vi "Flow Cal_Buffer_Dbl_VIG.vi"(0 "Fuel Temp":dbl, 1 "Operation":T4(ring)=enum."set raw data", 3 "Constants":cluster{"Ti":dbl, "SGi":dbl}, 5 "Calibration Formulas":T3, 9 "Flow (GPM)":dbl, 11 "error in":errorcluster, 12 "SGH20":dbl, 14 "Valid Flow Ranges":dbl[](array[numeric])) -> (4 "Addtional Values":T2, 6 "Current Formulas":T3, 10 "Calibrated Flow (lb/hr)":dbl, 15 "error out":errorcluster)   [LabVIEW 2018]
uses:
  Common/Controls/Parsed Formula TDEF.ctl
  <vilib>/gmath/NI_Gmath.lvlib
panel:
  in  "Calibration Info":T1
  out "Parsed Formula":cluster{"Table":i32[][], "Y Values":dbl[]}
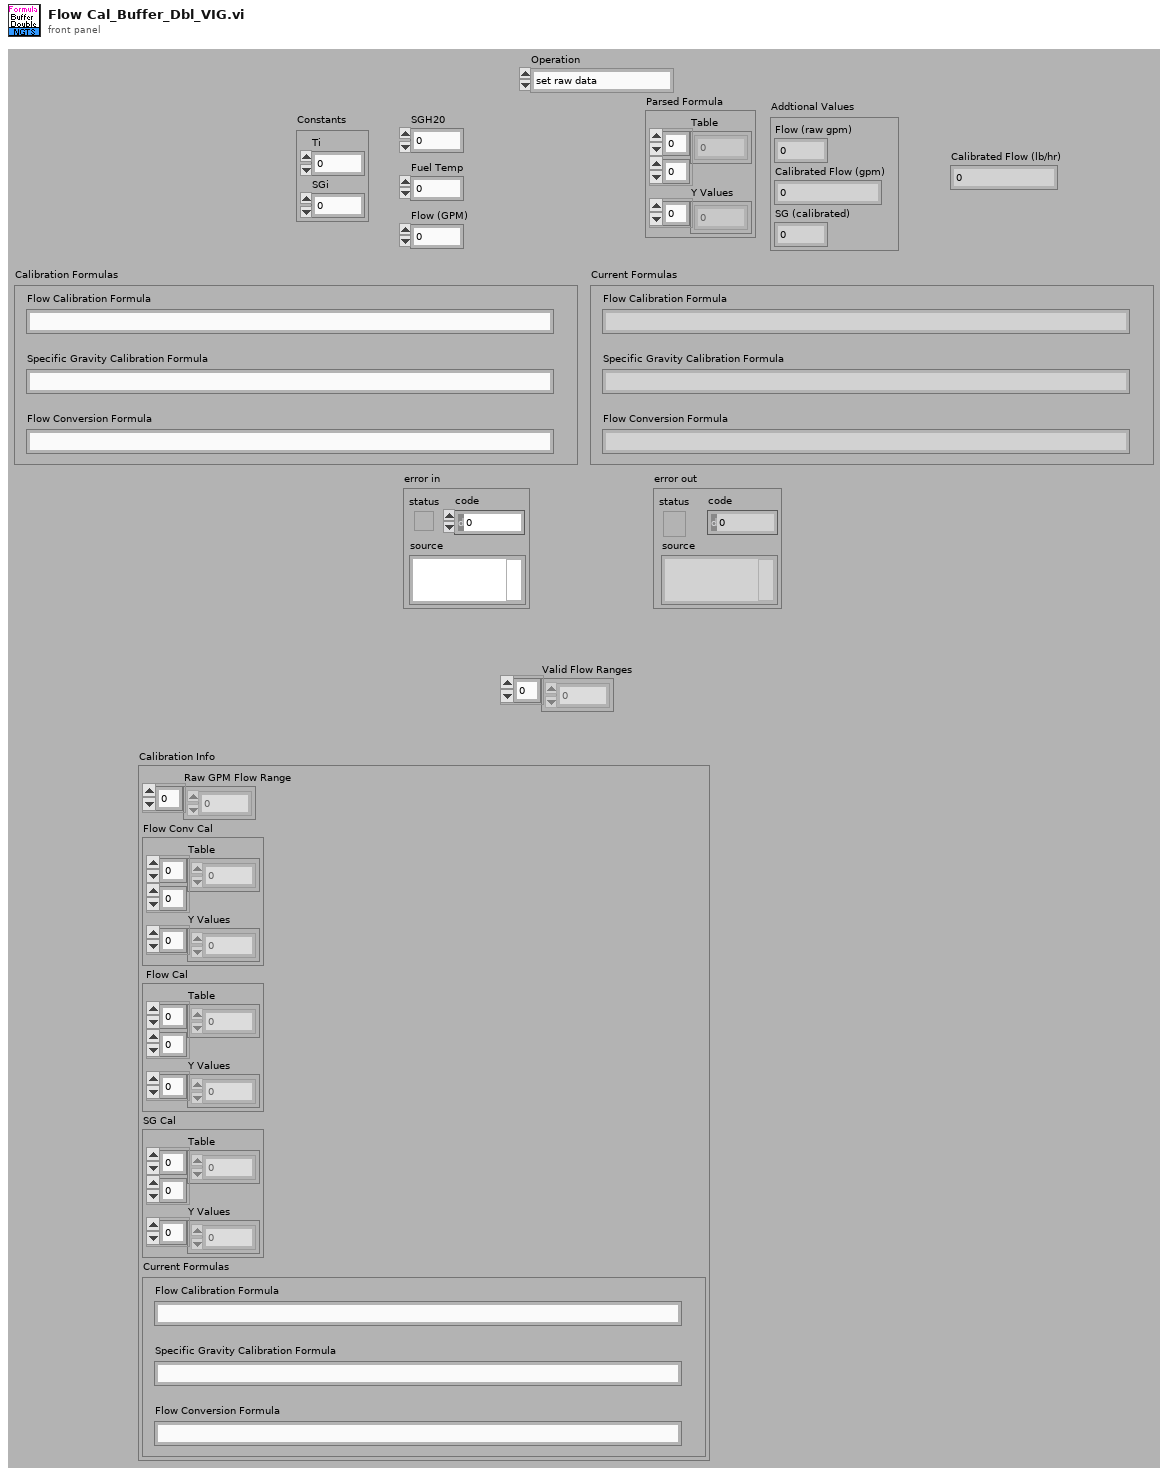
[diagram p1: front panel]
types:
  T1 = typedef "Parsed Formula TDEF.ctl" = cluster{"Raw GPM Flow Range":dbl[], "Flow Conv Cal":cluster{"Table":i32[][], "Y Values":dbl[]}, " Flow Cal":cluster{"Table":i32[][], "Y Values":dbl[]}, "SG Cal":cluster{"Table":i32[][], "Y Values":dbl[]}, "Current Formulas":cluster{"Flow Calibration Formula":string, "Specific Gravity Calibration Formula":string, "Flow Conversion Formula":string}}
  T2 = cluster{"Flow (raw gpm)":dbl, "Calibrated Flow (gpm)":dbl, "SG (calibrated)":dbl}
  T3 = cluster{"Flow Calibration Formula":string, "Specific Gravity Calibration Formula":string, "Flow Conversion Formula":string}
  T4 = enum16{"get data", "set raw data", "Set Ti and SGi and SGH20", "Add New Formula", "Get Formula", "initialize"}
  T5 = cluster{"element":dbl, "Flow (GPM)":dbl, "y value":dbl}
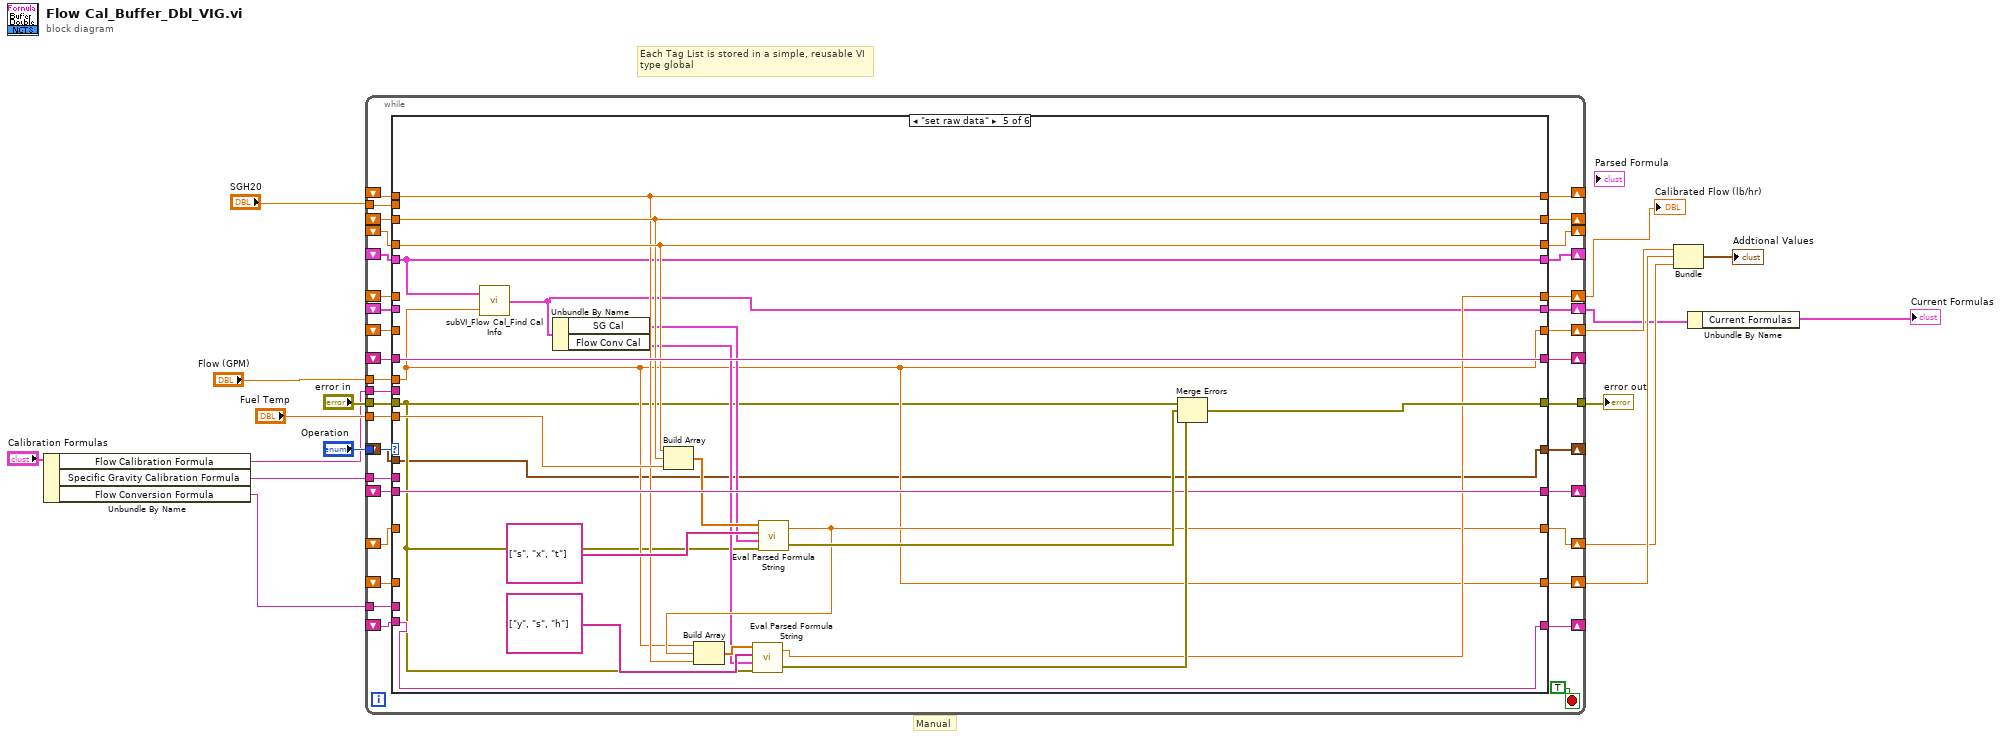
[diagram p0: block diagram]
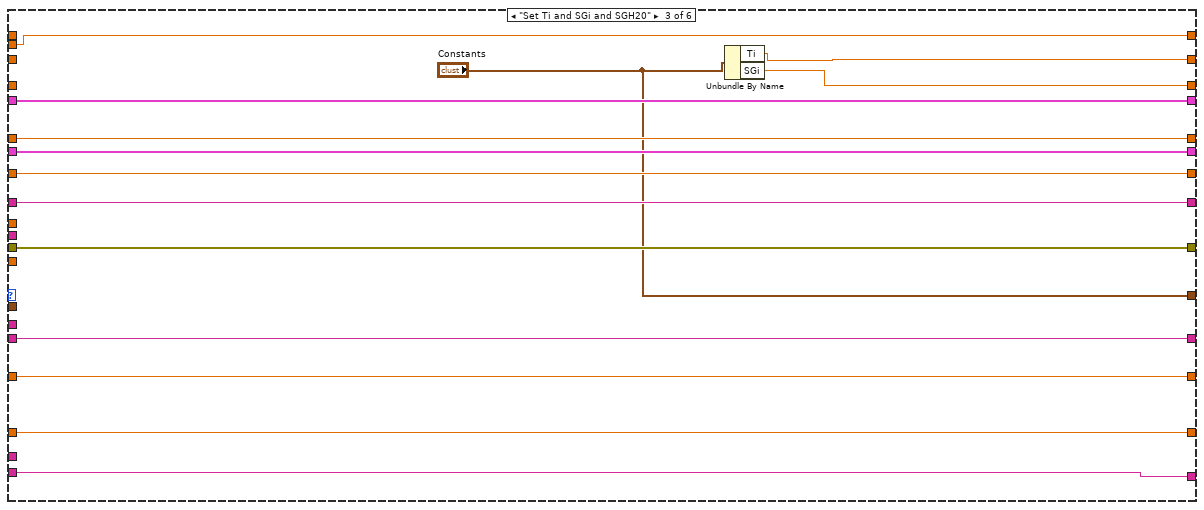
[diagram p4: hidden frame]
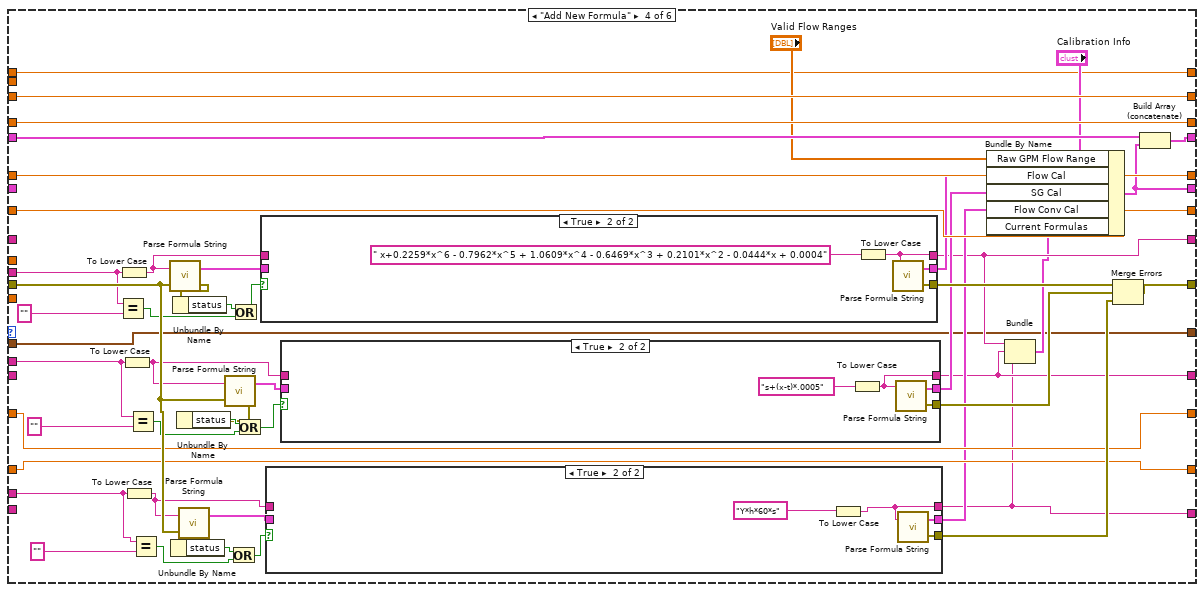
[diagram p5: hidden frame]
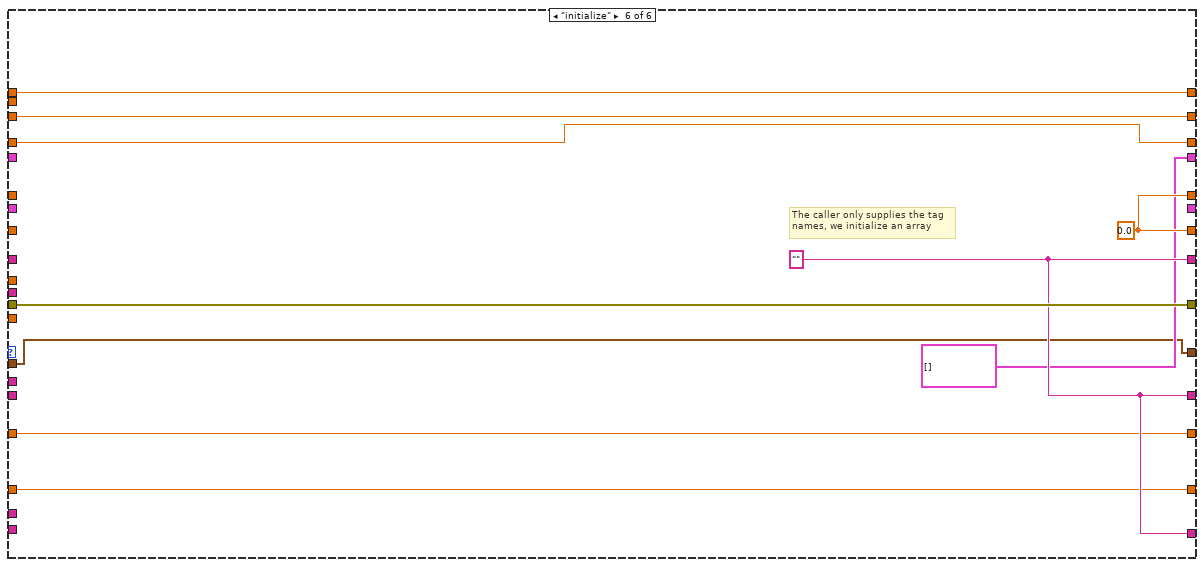
[diagram p9: hidden frame]
diagram:
  # "Manual"
  # "Each Tag List is stored in a simple, reusable VI\ntype global"
  n1 = Unbundle By Name("Calibration Formulas") -> ("Flow Calibration Formula"=w11:string, "Specific Gravity Calibration Formula"=w10:string, "Flow Conversion Formula"=w9:string)
  n2 = while {
    tunnel: "Operation" -> [w53]
    tunnel: "Flow (GPM)" -> [w51]
    tunnel: "error in" -> [w50]
    tunnel: [w49] -> w14
    shift-right: [w48] -> w5
    shift-left: _ -> [w47]
    shift-right: [w46] -> w6
    shift-left: _ -> [w42]
    shift-right: [w45] -> _
    shift-left: _ -> [w43]
    tunnel: w11 -> [w44]
    tunnel: w10 -> [w41]
    tunnel: w9 -> [w38]
    shift-right: [w40] -> _
    shift-left: _ -> [w36]
    shift-right: [w39] -> _
    shift-left: _ -> [w37]
    shift-right: [w35] -> _
    shift-left: _ -> [w33]
    shift-right: [w34] -> _
    shift-left: _ -> [w32]
    tunnel: "Fuel Temp" -> [w31]
    shift-right: [w30] -> _
    shift-left: _ -> [w29]
    shift-right: [w28] -> w7
    shift-left: _ -> [w26]
    shift-right: [w27] -> w8
    shift-left: _ -> [w25]
    tunnel: "SGH20" -> [w24]
    shift-right: [w23] -> _
    shift-left: _ -> [w22]
    shift-right: [w21] -> w3
    shift-left: _ -> [w20]
    shift-right: [w19] -> _
    shift-left: _ -> [w18]
    stop <- TRUE stop-if-true
    n3 = case shown="\"set raw data\"" w53 {
      tunnel: w51 -> [_ _ _ _ w165 _]
      tunnel: w50 -> [w67 w81 w95 w139 w164 w195]
      tunnel: [w67 w81 w95 w138 w184 w195] -> w49
      tunnel: [w66 w80 w94 w144 w165 w194] -> w48
      tunnel: w47 -> [w66 w80 w94 w144 _ _]
      tunnel: [w64 w78 w92 w143 w171 w194] -> w46
      tunnel: [w65 w79 w93 w101 w185 w193] -> w45
      tunnel: w44 -> [_ _ _ w127 _ _]
      tunnel: w43 -> [w65 w79 w93 _ w185 _]
      tunnel: w42 -> [w64 w78 w92 w143 _ _]
      tunnel: w41 -> [_ _ _ w115 _ _]
      tunnel: [w62 w76 w90 w99 w180 w193] -> w40
      tunnel: [w63 w77 w91 w100 w181 w193] -> w39
      tunnel: w38 -> [_ _ _ w116 _ _]
      tunnel: w37 -> [w63 w77 w91 _ w181 _]
      tunnel: w36 -> [w62 w76 w90 _ w180 _]
      tunnel: [w61 w75 w87 w131 w177 w192] -> w35
      tunnel: [w60 w74 w86 w130 w178 w191] -> w34
      tunnel: w33 -> [w61 w75 _ w131 w177 w192]
      tunnel: w32 -> [w60 w74 _ w130 w178 w191]
      tunnel: w31 -> [_ _ _ _ w176 _]
      tunnel: [w59 w73 w84 w102 w173 w190] -> w30
      tunnel: w29 -> [w59 w73 _ w102 w173 w190]
      tunnel: [w58 w72 w89 w129 w170 w189] -> w28
      tunnel: [w57 w71 w88 w128 w165 w188] -> w27
      tunnel: w26 -> [w58 w72 w89 w129 _ w189]
      tunnel: w25 -> [w57 w71 w88 w128 _ w188]
      tunnel: w24 -> [_ _ w84 _ _ _]
      tunnel: [w56 w70 w85 w108 w169 T1[] [] ("Calibration Parsed Formulas")] -> w23
      tunnel: w22 -> [w56 w70 w85 w109 w169 _]
      tunnel: [w55 w69 w83 w97 w166 _] -> w21
      tunnel: w20 -> [w55 w69 w83 _ _ _]
      tunnel: [w54 w68 "Constants" w96 w163 w186] -> w19
      tunnel: w18 -> [w54 w68 _ w96 w163 w186]
      frame "get data", Default {
      }
      frame "Get Formula" {
      }
      frame "Set Ti and SGi and SGH20" {
        n4 = Unbundle By Name("Constants") -> ("Ti"=w87:dbl, "SGi"=w86:dbl)
      }
      frame "Add New Formula" {
        n5 = Equal?(x=w127, y="") -> (x = y?=w125:bool)
        n6 = To Lower Case(string=w127) -> (all lower case string=w140:string)
        n7 = To Lower Case(string=w115) -> (all lower case string=w134:string)
        n8 = To Lower Case(string=w116) -> (all lower case string=w133:string)
        n9 = Equal?(x=w115, y="") -> (x = y?=w113:bool)
        n10 = Equal?(x=w116, y="") -> (x = y?=w114:bool)
        n11 = call <vilib>:"Parse Formula String.vi"("error in (no error)"=w139, "formula"=w140) -> ("error out"=w123:errorcluster, "Parsed Formula"=w141:cluster{"Table":i32[][], "Y Values":dbl[]})
        n12 = Unbundle By Name(w123) -> ("status"=w122:bool)
        n13 = call <vilib>:"Parse Formula String.vi"("error in (no error)"=w139, "formula"=w133) -> ("error out"=w111:errorcluster, "Parsed Formula"=w132:cluster{"Table":i32[][], "Y Values":dbl[]})
        n14 = Unbundle By Name(w111) -> ("status"=w120:bool)
        n15 = call <vilib>:"Parse Formula String.vi"("error in (no error)"=w139, "formula"=w134) -> ("error out"=w112:errorcluster, "Parsed Formula"=w135:cluster{"Table":i32[][], "Y Values":dbl[]})
        n16 = Unbundle By Name(w112) -> ("status"=w121:bool)
        n17 = Or(x=w120, y=w114) -> (x .or. y?=w110:bool)
        n18 = Or(x=w122, y=w125) -> (x .or. y?=w124:bool)
        n19 = Or(x=w121, y=w113) -> (x .or. y?=w119:bool)
        n20 = case shown="True" w124 {
          tunnel: [_ w162] -> w142
          tunnel: [w158 w161] -> w105
          tunnel: w141 -> [w158 _]
          tunnel: [w157 w160] -> w101
          tunnel: w140 -> [w157 _]
          frame False {
          }
          frame True {
            n21 = To Lower Case(string=" x+0.2259*x^6 - 0.7962*x^5 + 1.0609*x^4 - 0.6469*x^3 + 0.2101*x^2 - 0.0444*x + 0.0004" ("formula")) -> (all lower case string=w160:string)
            n22 = call <vilib>:"Parse Formula String.vi"("formula"=w160) -> ("error out"=w162:errorcluster, "Parsed Formula"=w161:cluster{"Table":i32[][], "Y Values":dbl[]})  [unwired: 1 in]
          }
        }
        n23 = case shown="True" w110 {
          tunnel: [_ w150] -> w136
          tunnel: [w146 w149] -> w104
          tunnel: w132 -> [w146 _]
          tunnel: [w145 w147] -> w99
          tunnel: w133 -> [w145 _]
          frame False {
          }
          frame True {
            n24 = To Lower Case(string="Y*h*60*s" ("formula")) -> (all lower case string=w147:string)
            n25 = call <vilib>:"Parse Formula String.vi"("formula"=w147) -> ("error out"=w150:errorcluster, "Parsed Formula"=w149:cluster{"Table":i32[][], "Y Values":dbl[]})  [unwired: 1 in]
          }
        }
        n26 = case shown="True" w119 {
          tunnel: [_ w156] -> w137
          tunnel: [w152 w155] -> w103
          tunnel: w135 -> [w152 _]
          tunnel: [w151 w153] -> w100
          tunnel: w134 -> [w151 _]
          frame False {
          }
          frame True {
            n27 = To Lower Case(string="s+(x-t)*.0005" ("formula")) -> (all lower case string=w153:string)
            n28 = call <vilib>:"Parse Formula String.vi"("formula"=w153) -> ("error out"=w156:errorcluster, "Parsed Formula"=w155:cluster{"Table":i32[][], "Y Values":dbl[]})  [unwired: 1 in]
          }
        }
        n29 = Bundle(w101, w100, w99) -> (w98:cluster{string, string, string})  [unwired: 1 in]
        n30 = Bundle By Name(cluster="Calibration Info", "Raw GPM Flow Range"="Valid Flow Ranges", "Flow Cal"=w105, "SG Cal"=w103, "Flow Conv Cal"=w104, "Current Formulas"=w98) -> (w97:T1)
        n31 = Merge Errors(w142, w137, w136) -> (w138:errorcluster)
        n32 = Build Array (concatenate)(w109, w97) -> (w108:T1[])
      }
      frame "set raw data" {
        n33 = call "subVI_Flow Cal_Find Cal Info.vi"("Flow (raw GPM)"=w165, "Calibration Parsed Formulas"=w169) -> ("Calibration Info"=w166:T1)
        n34 = Unbundle By Name(w166) -> ("SG Cal"=w168:cluster{"Table":i32[][], "Y Values":dbl[]}, "Flow Conv Cal"=w167:cluster{"Table":i32[][], "Y Values":dbl[]})
        n35 = Build Array(w178, w177, w176) -> (w175:dbl[])
        n36 = call <vilib>:"Eval Parsed Formula String.vi"("error in (no error)"=w164, "Parsed Formula"=w168, "Variables"=string[] ["s", "x", "t"], "X Values"=w175) -> ("error out"=w183:errorcluster, "y value"=w170:dbl)
        n37 = Build Array(w165, w170, w173) -> (w174:dbl[])
        n38 = call <vilib>:"Eval Parsed Formula String.vi"("error in (no error)"=w164, "Parsed Formula"=w167, "Variables"=string[] ["y", "s", "h"], "X Values"=w174) -> ("error out"=w182:errorcluster, "y value"=w171:dbl)
        n39 = Merge Errors(w164, w183, w182) -> (w184:errorcluster)
      }
      frame "initialize" {
        w193 = "" ("String")
        w194 = 0.0 ("element")
        # "The caller only supplies the tag\nnames, we initialize an array"
      }
    }
  }
  "error out" <- w14
  "Calibrated Flow (lb/hr)" <- w6
  n40 = Bundle("element"=w5, "Flow (GPM)"=w8, "y value"=w7) -> (→"Addtional Values":T5)  [unwired: 1 in]
  n41 = Unbundle By Name(w3) -> ("Current Formulas"=→"Current Formulas":T3)
